vi "Write Drink Type.vi"(8 "error in (no error)":errorcluster, 10 "Drink Type":T1, 11 "Beverage in":refnum<class "Beverage.lvclass">) -> (0 "error out":errorcluster, 3 "Beverage out":refnum<class "Beverage.lvclass">)   [LabVIEW 2023, in "Beverage.lvclass"]
doc: "Simple accessor method to set the <b>Drink Type</b> of a Beverage."
uses:
  Beverage.lvclass
  TypeDefs/Drink Type.ctl
  Beverage.lvclass/Beverage.ctl
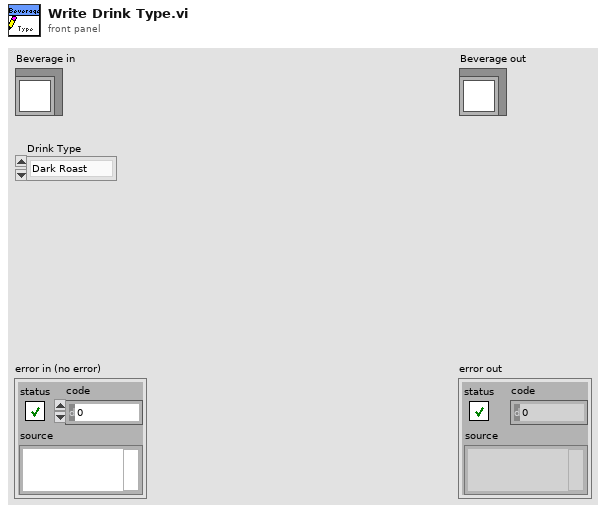
[diagram p1: front panel]
types:
  T1 = typedef "Beverage.lvclass/Drink Type.ctl" = enum16{"Dark Roast", "Decaf", "Espresso", "House Blend"}
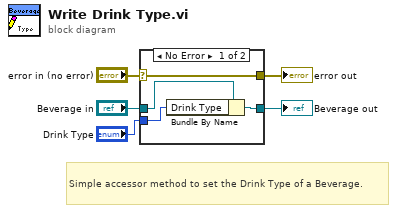
[diagram p0: block diagram]
diagram:
  # "Simple accessor method to set the Drink Type of a Beverage."
  n1 = case shown="No Error" "error in (no error)" {
    selector: "error in (no error)" -> [w9 w10]
    tunnel: [w9 w10] -> w4
    tunnel: [w7 w11] -> w2
    tunnel: "Beverage in" -> [w8 w11]
    tunnel: "Drink Type" -> [w6 _]
    frame No Error {
      n2 = Bundle By Name(cluster=w8, "Drink Type"=w6) -> (w7:refnum<class "Beverage.lvclass">)
    }
    frame Error {
    }
  }
  "error out" <- w4
  "Beverage out" <- w2
